vi "Anritsu VNA Read Learn String.vi"(7 "Anritsu VNA":T1, 8 "error in (no error)":errorcluster, 11 "VISA Resource Name":refnum<visa-resource-name>) -> (0 "error out":errorcluster, 2 "Learn String":string, 3 "dup VISA Resource Name":refnum<visa-resource-name>)   [LabVIEW 2011]
uses:
  TypeDefs/Anritsu VNA Instrument Info.ctl
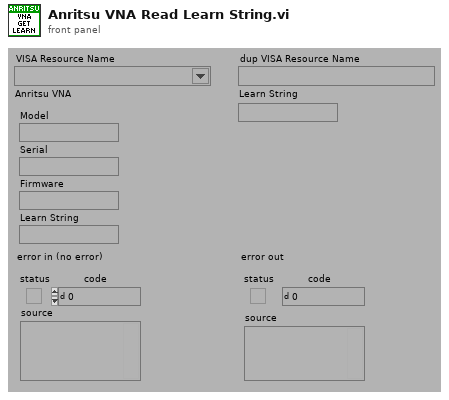
[diagram p1: front panel]
types:
  T1 = typedef "Anritsu VNA Instrument Info.ctl" = cluster{"Model":string, "Serial":string, "Firmware":string, "Learn String":string}
  T2 = typedef "Anritsu VNA Model.ctl" = enum16{"Not Supported", "37XXXX", "MS20XXX", "MS462XX", "MS464XX"}
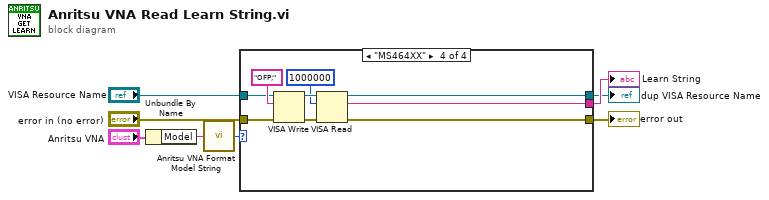
[diagram p0: block diagram]
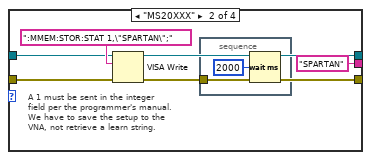
[diagram p3: hidden frame]
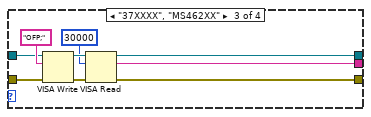
[diagram p4: hidden frame]
diagram:
  n1 = Unbundle By Name("Anritsu VNA") -> ("Model"=w1:string)
  n2 = call "Anritsu VNA Format Model String.vi"("Model"=w1) -> ("Model"=w3:T2)
  n3 = case shown="\"MS464XX\"" w3 {
    tunnel: "VISA Resource Name" -> [w9 w15 w25 w34]
    tunnel: [_ "SPARTAN" w19 w28] -> w7
    tunnel: "error in (no error)" -> [w10 w14 w24 w33]
    tunnel: [w10 w11 w21 w30] -> w5
    tunnel: [w9 w13 w20 w29] -> w4
    frame "Not Supported" {
    }
    frame "MS20XXX" {
      # "A 1 must be sent in the integer\nfield per the programmer's manual.\nWe have to save the setup to the\nVNA, not retrieve a learn string."
      n4 = VISA Write(VISA resource name=w15, write buffer=":MMEM:STOR:STAT 1,\"SPARTAN\";", error in (no error)=w14) -> (VISA resource name out=w13:refnum<visa-resource-name>, error out=w11:errorcluster)  [unwired: 1 out]
      n5 = stacked-sequence {
        tunnel: w11 -> [_]
        frame #0 {
          n6 = Wait (ms)(milliseconds to wait=u32 2000) -> ()  [unwired: 1 out]
        }
      }
    }
    frame "37XXXX", "MS462XX" {
      n7 = VISA Write(VISA resource name=w25, write buffer="OFP;", error in (no error)=w24) -> (VISA resource name out=w23:refnum<visa-resource-name>, error out=w22:errorcluster)  [unwired: 1 out]
      n8 = VISA Read(VISA resource name=w23, byte count=u32 30000, error in (no error)=w22) -> (VISA resource name out=w20:refnum<visa-resource-name>, read buffer=w19:string, error out=w21:errorcluster)  [unwired: 1 out]
    }
    frame "MS464XX" {
      n9 = VISA Write(VISA resource name=w34, write buffer="OFP;", error in (no error)=w33) -> (VISA resource name out=w32:refnum<visa-resource-name>, error out=w31:errorcluster)  [unwired: 1 out]
      n10 = VISA Read(VISA resource name=w32, byte count=u32 1000000, error in (no error)=w31) -> (VISA resource name out=w29:refnum<visa-resource-name>, read buffer=w28:string, error out=w30:errorcluster)  [unwired: 1 out]
    }
  }
  "error out" <- w5
  "dup VISA Resource Name" <- w4
  "Learn String" <- w7
